vi "Get Leave Open.vi"(11 "Processing in":refnum<class "Processing.lvclass">) -> (2 "Leave Open":bool, 3 "Processing out":refnum<class "Processing.lvclass">)   [LabVIEW 2020, in "HTTP Server.lvlib" / "Processing.lvclass"]
uses:
  Processing.lvclass
  Processing.lvclass/Processing.ctl
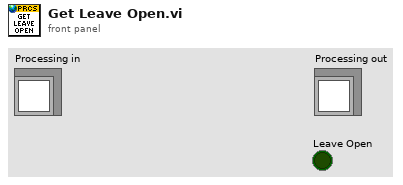
[diagram p1: front panel]
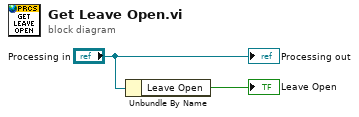
[diagram p0: block diagram]
diagram:
  n1 = Unbundle By Name("Processing in") -> ("Leave Open"=→"Leave Open":bool)
  "Processing out" <- "Processing in"
